vi "SaveData01.vi"(6 "Dupicate":bool, 7 "Index Row":i32, 9 "Save Data In":string[](array[string]), 10 "DataTable In":string[][](array[string]), 11 "file path (dialog if empty)":path) -> (1 "Save Data Out":string[](array[string]), 2 "DataTable Out":string[][](array[string]))   [LabVIEW 2014]
uses:
  <vilib>/Utility/file.llb/Write To Spreadsheet File (string).vi
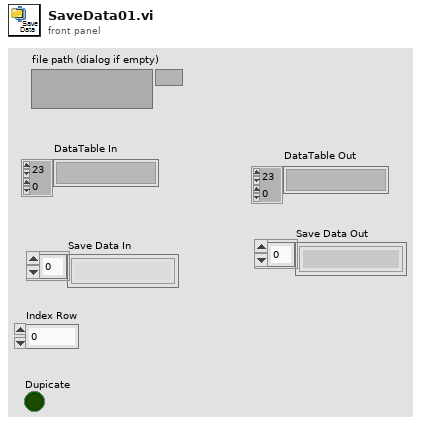
[diagram p1: front panel]
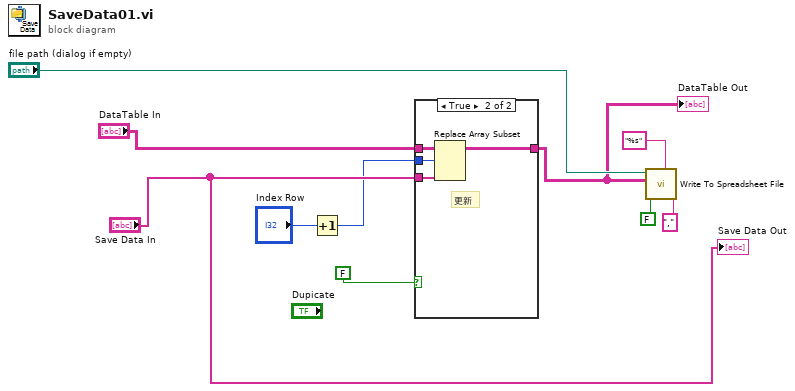
[diagram p0: block diagram]
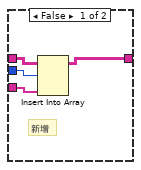
[diagram p2: hidden frame]
diagram:
  n1 = Increment(x="Index Row") -> (x+1=w2:i32)
  n2 = case shown="True" FALSE {
    tunnel: "DataTable In" -> [w14 w18]
    tunnel: "Save Data In" -> [w11 w17]
    tunnel: w2 -> [w12 w16]
    tunnel: [w13 w15] -> w5
    frame False {
      # "新增"
      n3 = Insert Into Array "Insert Into Array"(array=w14, index (row)=w12, new element=w11) -> (w13:string[][])  [unwired: 1 in]
    }
    frame True {
      # "更新"
      n4 = Replace Array Subset(array=w18, new element=w17, index (row)=w16) -> (w15:string[][])  [unwired: 1 in]
    }
  }
  "DataTable Out" <- w5
  n5 = call-poly <vilib>:"Write To Spreadsheet File.vi"("delimiter (\\t)"="," ("delimiter (\\t)"), "format (%s)"="%s", "append to file? (new file:F)"=FALSE, "2D data"=w5, "file path (dialog if empty)"="file path (dialog if empty)") -> ()  [unwired: 3 in, 1 out]
  "Save Data Out" <- "Save Data In"
